vi "grab with palette options.vi"() -> ()   [LabVIEW 2013]
panel:
  in  "Palette:Palette Type":u32(ring) items=["Grayscale", "Binary", "Gradient", "Rainbow", "Temperature", "User Defined"]
  out "ms between image":u32
  out "Frame Rate":dbl
  in  "Stop (F)":bool
  out "Image Out":T1(plugin-control)
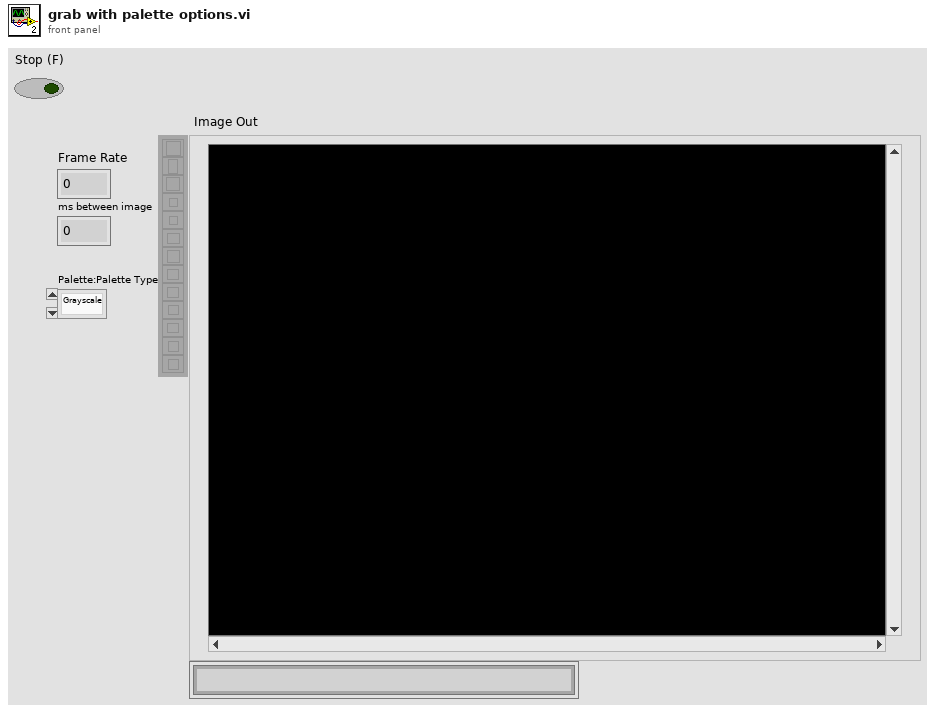
[diagram p1: front panel]
types:
  T1 = typedef "IMAQ Image.ctl" = refnum<image>
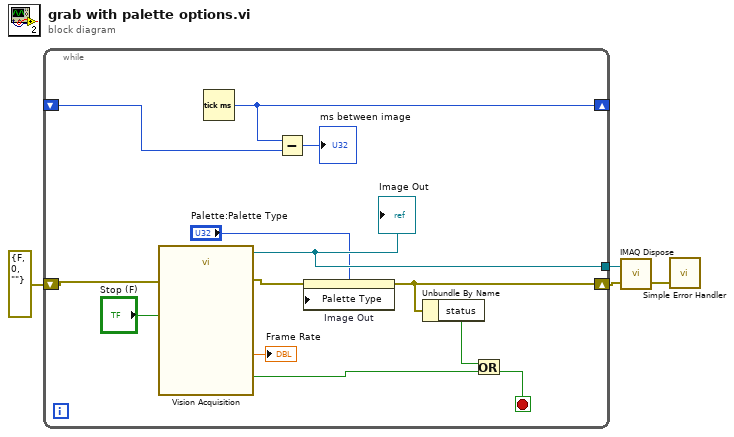
[diagram p0: block diagram]
diagram:
  n1 = while {
    shift-right: [w14] -> _
    shift-left: _ -> [w13]
    shift-right: [w7] -> w4
    shift-left: errorcluster {"status"=FALSE, "code"=0, "source"=""} ("error out") -> [w10]
    tunnel: [w9] -> w2
    stop <- w11 stop-if-true
    n2 = call "Vision Acquisition"("Stop (F)"="Stop (F)", "error in"=w10) -> ("Image Out"=w9:T1, "Frame Rate"=→"Frame Rate":dbl, "Stopped"=w16:bool, "error out"=w8:errorcluster)  [unwired: 22 in]
    "Image Out" <- w9
    n3 = Tick Count (ms)() -> (millisecond timer value=w14:u32)
    n4 = Subtract(x=w14, y=w13) -> (x-y=→"ms between image":u32)
    n5 = property on="Image Out" class="ImageControl"(error in=w8, "Palette Type"="Palette:Palette Type") -> (error out=w7:errorcluster)  [unwired: 1 in, 1 out]
    n6 = Unbundle By Name(w7) -> ("status"=w6:bool)
    n7 = Or(x=w6, y=w16) -> (x .or. y?=w11:bool)
  }
  n8 = call "IMAQ Dispose"("Image"=w2, "error in (no error)"=w4) -> ("error out"=w1:errorcluster)  [unwired: 4 in]
  n9 = call <vilib>:"Simple Error Handler.vi"("error in (no error)"=w1) -> ()  [unwired: 4 in, 5 out]
